vi "Sentran Accuracy Test SAA.vi"(8 "error in (no error)":errorcluster, 10 "Model in":refnum<class "Model.lvclass">, 11 "Test Actuator State in":refnum<class "Test Actuator State.lvclass">) -> (0 "error out":errorcluster, 2 "Model out":refnum<class "Model.lvclass">, 3 "Test Actuator State out":refnum<class "Test Actuator State.lvclass">)   [LabVIEW 2016, in "Test Actuator State.lvclass"]
uses:
  Test Actuator State.lvclass
  Model/Model/Model.lvclass
  Model/Model/Model.lvclass/Model.ctl
  Typedefs/ActuatorSetPoints.ctl
  <vilib>/Platform/TimedLoop/XDataNode/timing_clust.ctl
  <vilib>/Platform/TimedLoop/XDataNode/nitl_modes.ctl
  <vilib>/Platform/TimedLoop/XDataNode/wakeup.ctl
  <vilib>/platform/TimedLoop/XDataNode/XDataNode.xnode
  Typedefs/FAMT Typedefs.lvlib
  <vilib>/Platform/TimedLoop/XDataNode/XDNodeRunTimeDep.lvlib
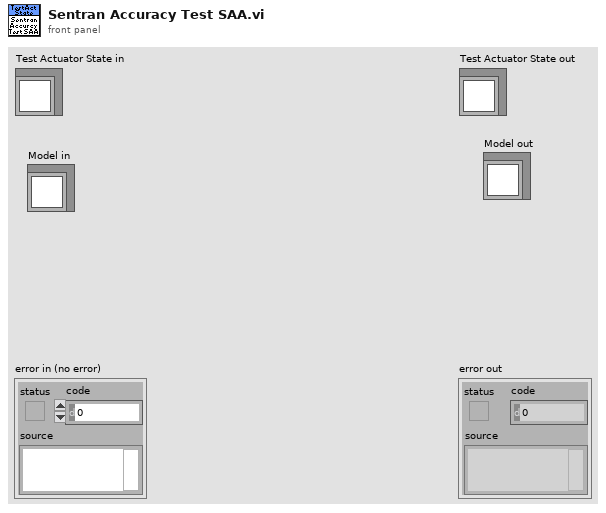
[diagram p1: front panel]
types:
  T1 = typedef "FAMT Typedefs.lvlib/SentranAccuracyTestSettings.ctl" = cluster{"Force Tolerance (N)":dbl, "Force Modifies (%)":dbl[], "Process Time (s)":dbl, "Sample Time (s)":dbl, "Max Moment (NM)":dbl}
  T2 = typedef "FAMT Typedefs.lvlib/FullForceScanSettings.ctl" = cluster{"Force Tolerance (N)":dbl, "DAA Force Set Points":T3[], "Process Time (s)":dbl, "Sample Time (s)":dbl, "Max Moment (NM)":dbl, "SAA Force Set Points":T3[]}
  T3 = typedef "FAMT Typedefs.lvlib/ForcePair.ctl" = cluster{"Axial Force":dbl, "Lateral Force":dbl}
  T4 = typedef "FAMT Typedefs.lvlib/ActuatorSetPoints.ctl" = cluster{"Axial Force":dbl, "Lateral Force":dbl, "FC1 Force":dbl, "FC2 Force":dbl}
  T5 = typedef "XDNodeRunTimeDep.lvlib/timing_clust.ctl" = cluster{"Expected End [f-1]":u64, "Actual End [f-1]":u64, "Finished Late? [f-1]":bool, "Expected End [i-1]":u64, "Actual End [i-1]":u64, "Finished Late? [i-1]":bool, "Expected Start [i]":u64, "Actual Start [i]":u64, "Expected Start [f]":u64, "Actual Start [f]":u64, "Source Name":string, "Structure Name":string, "Period":i64, "Deadline":i64, "Offset":i64, "Start":i64, "Priority":i32, "Timeout":i32, "Mode":T6, "Wakeup Reason":T7, "Error":errorcluster, "Source Type":string, "Secondary Source Type":string, "Global End Time":u64, "Global Start Time":u64, "Frame Duration":u64, "Iteration Duration":u64, "Assigned CPU":i32, "I/O Scan Engine Mode":u32}
  T6 = typedef "XDNodeRunTimeDep.lvlib/nitl_modes.ctl" = enum32{"No Change", "Process missed periods, maintain original phase", "Discard missed periods, maintain original phase", "Process missed periods, ignore original phase", "Discard missed periods, ignore original phase"}
  T7 = typedef "XDNodeRunTimeDep.lvlib/wakeup.ctl" = enum32{"Normal", "Aborted", "Asynchronous wakeup", "Timing source error", "Timed loop error", "Timeout"}
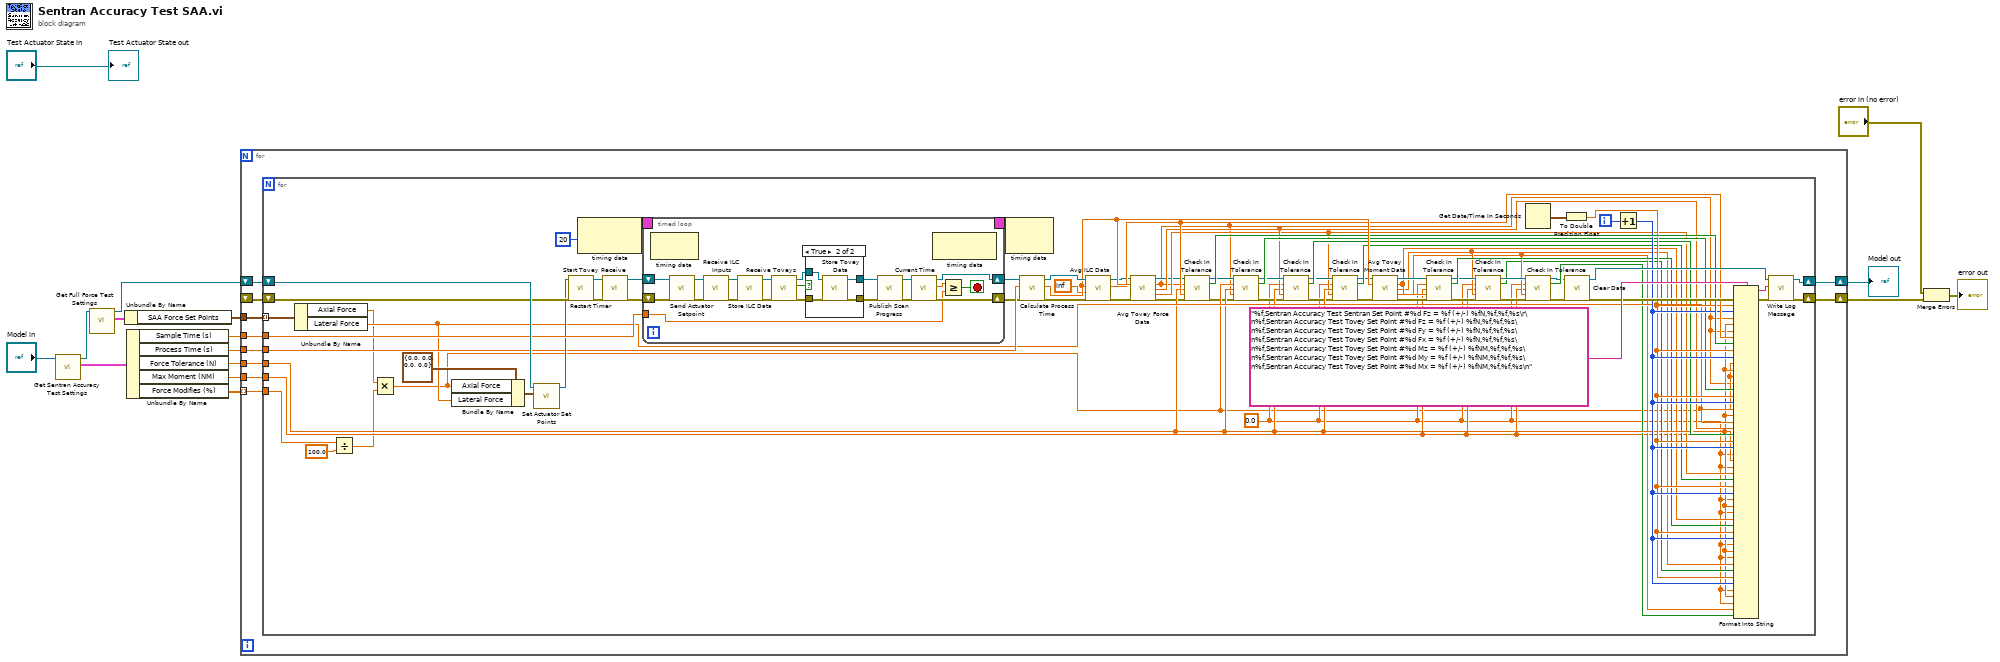
[diagram p0: block diagram]
diagram:
  n1 = call "Get Sentran Accuracy Test Settings.vi"("Model in"="Model in") -> ("Sentran Accuracy Test Settings"=w7:T1, "Model out"=w1:refnum<class "Model.lvclass">)  [unwired: 9 in]
  n2 = call "Get Full Force Test Settings.vi"("Model in"=w1) -> ("Full Force Test Settings"=w10:T2, "Model out"=w15:refnum<class "Model.lvclass">)  [unwired: 9 in]
  n3 = Unbundle By Name(w10) -> ("SAA Force Set Points"=w9:T3[])
  n4 = Unbundle By Name(w7) -> ("Sample Time (s)"=w6:dbl, "Process Time (s)"=w5:dbl, "Force Tolerance (N)"=w4:dbl, "Max Moment (NM)"=w3:dbl, "Force Modifies (%)"=w2:dbl[])
  n5 = for {
    tunnel: w9 -> [w23]
    tunnel: w6 -> [w22]
    tunnel: w5 -> [w21]
    tunnel: w4 -> [w20]
    tunnel: w3 -> [w19]
    shift-right: [w25] -> w12
    shift-left: w15 -> [w26]
    shift-right: [w24] -> w11
    shift-left: _ -> [w18]
    tunnel: w2 -> [w17] mode=indexing
    n6 = for {
      tunnel: w23 -> [w86] mode=indexing
      shift-right: [w96] -> w25
      shift-left: w26 -> [w100]
      tunnel: w22 -> [w99]
      tunnel: w21 -> [w81]
      tunnel: w20 -> [w65]
      shift-right: [w82] -> w24
      shift-left: w18 -> [w98]
      tunnel: w19 -> [w44]
      tunnel: w17 -> [w41]
      i -> [w93]
      w43 = 0.0
      n7 = Unbundle By Name(w86) -> ("Axial Force"=w38:dbl, "Lateral Force"=w69:dbl)
      n8 = Divide(x=w41, y=100.0) -> (x/y=w39:dbl)
      n9 = Multiply(x=w38, y=w39) -> (x*y=w37:dbl)
      n10 = Bundle By Name(cluster=T4 {"Axial Force"=0.0, "Lateral Force"=0.0, "FC1 Force"=0.0, "FC2 Force"=0.0} ("Actuator Set Points"), "Axial Force"=w37, "Lateral Force"=w69) -> (w87:T4)
      n11 = call "Set Actuator Set Points.vi"("Actuator Set Points"=w87, "Model in"=w100) -> ("Model out"=w88:refnum<class "Model.lvclass">)  [unwired: 9 in]
      n12 = call "Restart Timer.vi"("error in (no error)"=w98, "Model in"=w88) -> ("error out"=w91:errorcluster, "Model out"=w92:refnum<class "Model.lvclass">)  [unwired: 8 in]
      n13 = node-c288(i64 20 ("Period")) -> (w29:T5)
      n14 = call "Start Tovey Receive.vi"("error in (no error)"=w91, "Model in"=w92) -> ("error out"=w89:errorcluster, "Model out"=w90:refnum<class "Model.lvclass">)  [unwired: 8 in]
      n15 = timed-loop {
        shift-right: [w115] -> w80
        shift-left: w90 -> [w121]
        shift-right: [w114] -> w78
        shift-left: w89 -> [w118]
        tunnel: w99 -> [w112]
        timing: w29 -> [_]
        timing-out: [_] -> w28
        stop <- w111 stop-if-true
        n16 = node-c288() -> ()  [unwired: 1 in, 1 out]
        n17 = call "Send Actuator Setpoint.vi"("error in (no error)"=w118, "Model in"=w121) -> ("error out"=w117:errorcluster, "Model out"=w120:refnum<class "Model.lvclass">)  [unwired: 8 in]
        n18 = call "Receive ILC Inputs.vi"("error in (no error)"=w117, "Model in"=w120) -> ("error out"=w116:errorcluster, "Model out"=w119:refnum<class "Model.lvclass">)  [unwired: 8 in]
        n19 = call "Store ILC Data.vi"("error in (no error)"=w116, "Model in"=w119) -> ("error out"=w109:errorcluster, "Model out"=w110:refnum<class "Model.lvclass">)  [unwired: 8 in]
        n20 = call "Receive Toveys.vi"("error in (no error)"=w109, "Model in"=w110) -> ("error out"=w107:errorcluster, "Data Received"=w106:bool, "Model out"=w108:refnum<class "Model.lvclass">)  [unwired: 7 in]
        n21 = case shown="True" w106 {
          tunnel: w108 -> [w125 w129]
          tunnel: w107 -> [w124 w128]
          tunnel: [w124 w127] -> w102
          tunnel: [w125 w126] -> w105
          frame False {
          }
          frame True {
            n22 = call "Store Tovey Data.vi"("error in (no error)"=w128, "Model in"=w129) -> ("error out"=w127:errorcluster, "Model out"=w126:refnum<class "Model.lvclass">)  [unwired: 8 in]
          }
        }
        n23 = call "Publish Scan Progress.vi"("error in (no error)"=w102, "Model in"=w105) -> ("error out"=w103:errorcluster, "Model out"=w104:refnum<class "Model.lvclass">)  [unwired: 8 in]
        n24 = call "Current Time.vi"("error in (no error)"=w103, "Model in"=w104) -> ("error out"=w114:errorcluster, "Time"=w113:dbl, "Model out"=w115:refnum<class "Model.lvclass">)  [unwired: 7 in]
        n25 = node-c288() -> ()  [unwired: 1 in, 1 out]
        n26 = Greater Or Equal?(x=w113, y=w112) -> (x >= y?=w111:bool)
      }
      n27 = node-c288(w28) -> ()  [unwired: 1 out]
      n28 = call "Calculate Process Time.vi"("error in (no error)"=w78, "Seconds"=w81, "Model in"=w80) -> ("error out"=w77:errorcluster, "Time"=w76:dbl, "Model out"=w79:refnum<class "Model.lvclass">)  [unwired: 6 in]
      n29 = call "Avg ILC Data.vi"("error in (no error)"=w77, "Before This Time"=inf, "After This Time"=w76, "Model in"=w79) -> ("error out"=w33:errorcluster, "Fz"=w75:dbl, "Model out"=w36:refnum<class "Model.lvclass">)  [unwired: 4 in, 1 out]
      n30 = call "Avg Tovey Force Data.vi"("Model in"=w36, "After This Time"=w76, "error in (no error)"=w33) -> ("Model out"=w35:refnum<class "Model.lvclass">, "Fz"=w30:dbl, "Fy"=w67:dbl, "Fx"=w56:dbl, "error out"=w32:errorcluster)  [unwired: 8 in]
      n31 = call "Check In Tolerance.vi"("Model in"=w35, "Expected"=w30, "Tolerance"=w65, "Actual"=w75, "error in (no error)"=w32) -> ("Model out"=w34:refnum<class "Model.lvclass">, "Pass"=w74:bool, "error out"=w31:errorcluster)  [unwired: 8 in]
      n32 = call "Check In Tolerance.vi"("Model in"=w34, "Expected"=w37, "Tolerance"=w65, "Actual"=w30, "error in (no error)"=w31) -> ("Model out"=w70:refnum<class "Model.lvclass">, "Pass"=w71:bool, "error out"=w62:errorcluster)  [unwired: 8 in]
      n33 = call "Check In Tolerance.vi"("Model in"=w70, "Expected"=w43, "Tolerance"=w65, "Actual"=w67, "error in (no error)"=w62) -> ("Model out"=w66:refnum<class "Model.lvclass">, "Pass"=w68:bool, "error out"=w61:errorcluster)  [unwired: 8 in]
      n34 = call "Check In Tolerance.vi"("Model in"=w66, "Expected"=w43, "Tolerance"=w65, "Actual"=w56, "error in (no error)"=w61) -> ("Model out"=w59:refnum<class "Model.lvclass">, "Pass"=w64:bool, "error out"=w60:errorcluster)  [unwired: 8 in]
      n35 = call "Avg Tovey Moment Data.vi"("Model in"=w59, "After This Time"=w76, "error in (no error)"=w60) -> ("Model out"=w58:refnum<class "Model.lvclass">, "Mz"=w55:dbl, "My"=w52:dbl, "Mx"=w51:dbl, "error out"=w57:errorcluster)  [unwired: 8 in]
      n36 = call "Check In Tolerance.vi"("Model in"=w58, "Expected"=w43, "Tolerance"=w44, "Actual"=w55, "error in (no error)"=w57) -> ("Model out"=w54:refnum<class "Model.lvclass">, "Pass"=w63:bool, "error out"=w47:errorcluster)  [unwired: 8 in]
      n37 = call "Check In Tolerance.vi"("Model in"=w54, "Expected"=w43, "Tolerance"=w44, "Actual"=w52, "error in (no error)"=w47) -> ("Model out"=w53:refnum<class "Model.lvclass">, "Pass"=w50:bool, "error out"=w46:errorcluster)  [unwired: 8 in]
      n38 = Get Date/Time In Seconds() -> (seconds since 1Jan1904=w94:timestamp)
      n39 = call "Check In Tolerance.vi"("Model in"=w53, "Expected"=w43, "Tolerance"=w44, "Actual"=w51, "error in (no error)"=w46) -> ("Model out"=w48:refnum<class "Model.lvclass">, "Pass"=w49:bool, "error out"=w45:errorcluster)  [unwired: 8 in]
      n40 = To Double Precision Float(number=w94) -> (double precision float=w72:dbl)
      n41 = call "Clear Data.vi"("error in (no error)"=w45, "Model in"=w48) -> ("error out"=w84:errorcluster, "Model out"=w97:refnum<class "Model.lvclass">)  [unwired: 8 in]
      n42 = Increment(x=w93) -> (x+1=w73:i32)
      n43 = Format Into String(format string="%f,Sentran Accuracy Test Sentran Set Point #%d Fz = %f (+/-) %fN,%f,%f,%s\r\n%f,Sentran Accuracy Test Tovey Set Point #%d Fz = %f (+/-) %fN,%f,%f,%s\n%f,Sentran Accuracy Test Tovey Set Point #%d Fy = %f (+/-) %fN,%f,%f,%s\n%f,Sentran Accuracy Test Tovey Set Point #%d Fx = %f (+/-) %fN,%f,%f,%s\n%f,Sentran Accuracy Test Tovey Set Point #%d Mz = %f (+/-) %fNM,%f,%f,%s\n%f,Sentran Accuracy Test Tovey Set Point #%d My = %f (+/-) %fNM,%f,%f,%s\n%f,Sentran Accuracy Test Tovey Set Point #%d Mx = %f (+/-) %fNM,%f,%f,%s\n", error in=w84, w72, w73, w30, w65, w30, w75, w74, w72, w73, w37, w65, w37, w30, w71, w72, w73, w69, w65, w69, w67, w68, w72, w73, w43, w65, w43, w56, w64, w72, w73, w43, w44, w43, w55, w63, w72, w73, w43, w44, w43, w52, w50, w72, w73, w43, w44, w43, w51, w49) -> (resulting string=w85:string, error out=w83:errorcluster)  [unwired: 1 in]
      n44 = call "Write Log Message.vi"("error in (no error)"=w83, "Message"=w85, "Model in"=w97) -> ("error out"=w82:errorcluster, "Model out"=w96:refnum<class "Model.lvclass">)  [unwired: 7 in]
    }
  }
  "Model out" <- w12
  n45 = Merge Errors("error in (no error)", w11) -> (→"error out":errorcluster)
  "Test Actuator State out" <- "Test Actuator State in"
